vi "+and-5.vi"(1 "Input":dbl) -> (15 "Output Top":dbl, 17 "Output Low":dbl)   [LabVIEW 2014]
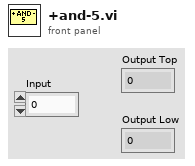
[diagram p1: front panel]
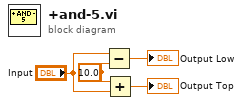
[diagram p0: block diagram]
diagram:
  w4 = 10.0
  n1 = Subtract(x="Input", y=w4) -> (x-y=→"Output Low":dbl)
  n2 = Add(x=w4, y="Input") -> (x+y=→"Output Top":dbl)
